vi "401_Add_Inspection_Audit_Data.vi"(0 "Current":variant, 1 "Previous":variant, 3 "Tolerance":u16(ring) items=["Area", "Width", "Height", "Spot", "Color", "Crack", "Foreign Particle", "Foreign outside Pocket"], 4 "Filter":u16(ring) items=["Area", "Width", "Height", "Smooth", "Solid"], 5 "Count":u16(ring) items=["Blister", "Blister 2", "OCV", "Splice 1", "Splice 2", "Pinhole 1", "Pinhole 2", "Spare Sensor 1", "Sealing", "OverPrinting", "Perforation", "Forming"], 7 "Error":errorcluster, 8 "Count/#Rej":string, 9 "Min/Max":string, 10 "Action":T1(ring), 11 "FilterMax/Min":string, 12 "Color":u16(ring) items=["Color 1", "Color 2"]) -> (27 "error out":errorcluster)   [LabVIEW 2015]
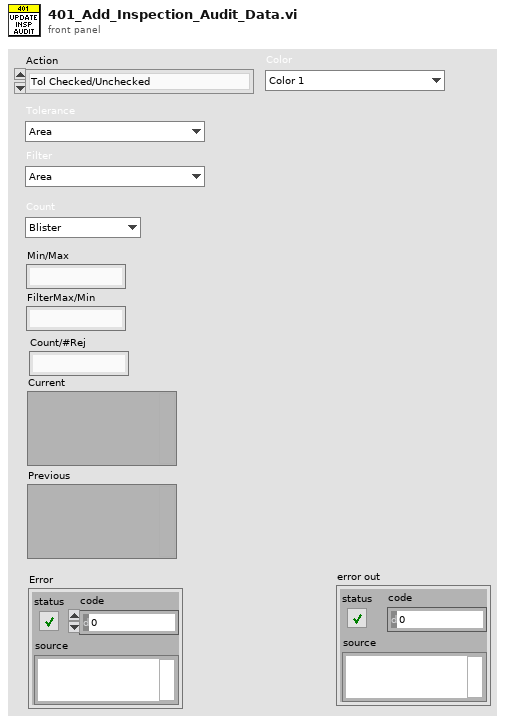
[diagram p1: front panel]
types:
  T1 = enum16{"Tol Checked/Unchecked", "Filter Checked/Unchecked", "Count Value updated", "Tol Updated", "Filter Updated"}
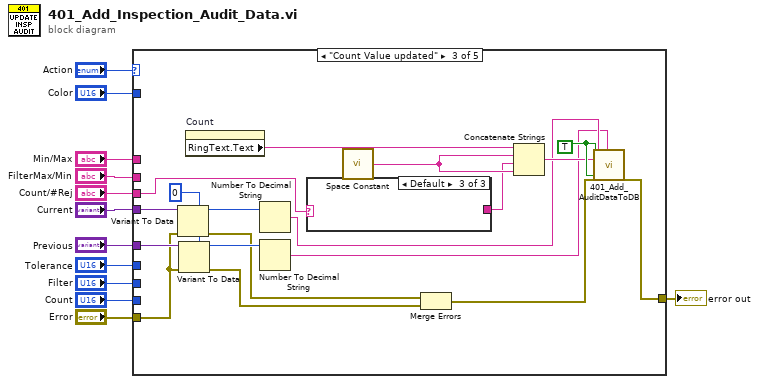
[diagram p0: block diagram]
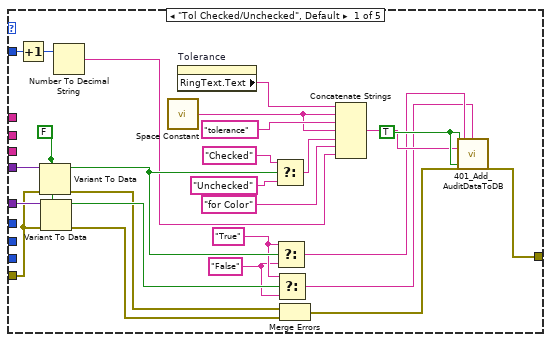
[diagram p2: hidden frame]
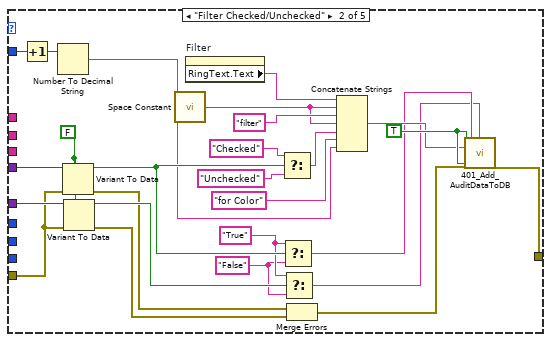
[diagram p3: hidden frame]
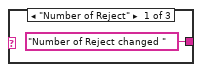
[diagram p4: hidden frame]
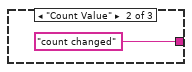
[diagram p5: hidden frame]
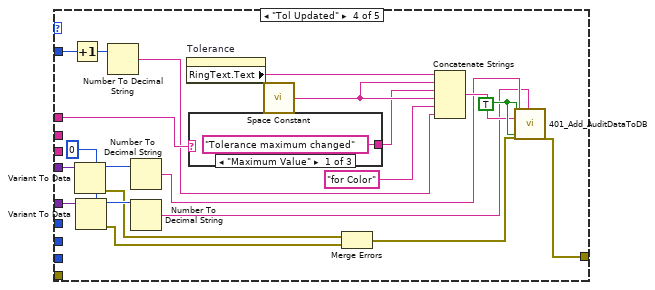
[diagram p6: hidden frame]
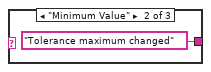
[diagram p7: hidden frame]
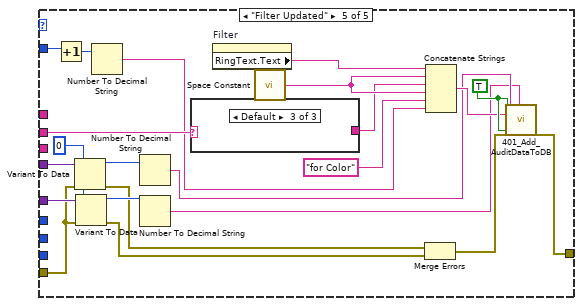
[diagram p9: hidden frame]
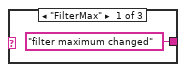
[diagram p10: hidden frame]
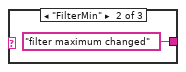
[diagram p11: hidden frame]
diagram:
  n1 = case shown="\"Count Value updated\"" "Action" {
    tunnel: "Current" -> [w38 w49 w78 w94 w118]
    tunnel: "Previous" -> [w37 w48 w77 w95 w119]
    tunnel: "Tolerance" -> [_ _ _ _ _]
    tunnel: "Filter" -> [_ _ _ _ _]
    tunnel: "Count" -> [_ _ _ _ _]
    tunnel: "FilterMax/Min" -> [_ _ _ _ w117]
    tunnel: "Min/Max" -> [_ _ _ w93 _]
    tunnel: "Error" -> [w21 w45 w70 _ w116]
    tunnel: [w17 w47 w66 w89 w112] -> w3
    tunnel: "Count/#Rej" -> [_ _ w65 _ _]
    tunnel: "Color" -> [w16 w41 _ w87 w109]
    frame "Tol Checked/Unchecked", Default {
      w24 = "False" ("string")
      w25 = "True" ("string")
      w29 = TRUE ("str(T)/num")
      w36 = FALSE
      n2 = Increment(x=w16) -> (x+1=w15:u16)
      n3 = Variant To Data(error in=w21, type=w36, Variant=w38) -> (data=w27:bool, error out=w19:errorcluster)
      n4 = Variant To Data(error in=w21, type=w36, Variant=w37) -> (data=w26:bool, error out=w18:errorcluster)
      n5 = Number To Decimal String(number=w15) -> (decimal integer string=w14:string)  [unwired: 1 in]
      n6 = call <vilib>:"Space Constant.vi"() -> ("String"=w33:string)
      n7 = property on="Tolerance" class="Ring (strict)"() -> ("RingText.Text"=w35:string)  [unwired: 2 in, 2 out]
      n8 = Select(t="Checked" ("string"), s=w27, f="Unchecked" ("string")) -> (s? t:f=w30:string)
      n9 = Select(t=w25, s=w27, f=w24) -> (s? t:f=w23:string)
      n10 = Select(t=w25, s=w26, f=w24) -> (s? t:f=w22:string)
      n11 = Merge Errors(w19, w18) -> (w20:errorcluster)
      n12 = Concatenate Strings(w35, w33, "tolerance" ("string"), w33, w30, "for Color" ("string"), w14) -> (w28:string)
      n13 = call "401_Add_AuditDataToDB.vi"("Str(T)/Num"=w29, "Activity"=w28, "Enum(F)/Str"=w29, "error in (no error)"=w20, "Current Value"=w23, "Previous Value"=w22) -> ("error out"=w17:errorcluster)  [unwired: 21 in]
    }
    frame "Filter Checked/Unchecked" {
      w52 = "False" ("string")
      w53 = "True" ("string")
      w57 = TRUE ("str(T)/num")
      w64 = FALSE
      n14 = Increment(x=w41) -> (x+1=w42:u16)
      n15 = Number To Decimal String(number=w42) -> (decimal integer string=w39:string)  [unwired: 1 in]
      n16 = Variant To Data(error in=w45, type=w64, Variant=w49) -> (data=w55:bool, error out=w44:errorcluster)
      n17 = Variant To Data(error in=w45, type=w64, Variant=w48) -> (data=w54:bool, error out=w43:errorcluster)
      n18 = call <vilib>:"Space Constant.vi"() -> ("String"=w61:string)
      n19 = property on="Filter" class="Ring (strict)"() -> ("RingText.Text"=w63:string)  [unwired: 2 in, 2 out]
      n20 = Select(t="Checked" ("string"), s=w55, f="Unchecked" ("string")) -> (s? t:f=w58:string)
      n21 = Select(t=w53, s=w55, f=w52) -> (s? t:f=w51:string)
      n22 = Select(t=w53, s=w54, f=w52) -> (s? t:f=w50:string)
      n23 = Merge Errors(w44, w43) -> (w46:errorcluster)
      n24 = Concatenate Strings(w63, w61, "filter" ("string"), w61, w58, "for Color" ("string"), w39) -> (w56:string)
      n25 = call "401_Add_AuditDataToDB.vi"("Str(T)/Num"=w57, "Activity"=w56, "Enum(F)/Str"=w57, "error in (no error)"=w46, "Current Value"=w51, "Previous Value"=w50) -> ("error out"=w47:errorcluster)  [unwired: 21 in]
    }
    frame "Count Value updated" {
      w76 = 0 ("Previous Value")
      w80 = TRUE ("str(T)/num")
      n26 = Variant To Data(error in=w70, type=w76, Variant=w78) -> (data=w75:i32, error out=w69:errorcluster)
      n27 = Variant To Data(error in=w70, type=w76, Variant=w77) -> (data=w73:i32, error out=w68:errorcluster)
      n28 = property on="Count" class="Ring (strict)"() -> ("RingText.Text"=w82:string)  [unwired: 2 in, 2 out]
      n29 = Number To Decimal String(number=w75) -> (decimal integer string=w72:string)  [unwired: 1 in]
      n30 = Number To Decimal String(number=w73) -> (decimal integer string=w71:string)  [unwired: 1 in]
      n31 = case shown="Default" w65 {
        tunnel: ["Number of Reject changed " ("string") "count changed" ("string") _] -> w74
        frame "Number of Reject" {
        }
        frame "Count Value" {
        }
        frame Default {
        }
      }
      n32 = call <vilib>:"Space Constant.vi"() -> ("String"=w81:string)
      n33 = Merge Errors(w69, w68) -> (w67:errorcluster)
      n34 = Concatenate Strings(w82, w81, w74, w81) -> (w79:string)
      n35 = call "401_Add_AuditDataToDB.vi"("Str(T)/Num"=w80, "Activity"=w79, "Enum(F)/Str"=w80, "error in (no error)"=w67, "Current Value"=w72, "Previous Value"=w71) -> ("error out"=w66:errorcluster)  [unwired: 21 in]
    }
    frame "Tol Updated" {
      w101 = 0 ("Previous Value")
      w103 = TRUE ("str(T)/num")
      n36 = Increment(x=w87) -> (x+1=w88:u16)
      n37 = Variant To Data(type=w101, Variant=w94) -> (data=w100:i32, error out=w92:errorcluster)  [unwired: 1 in]
      n38 = Variant To Data(type=w101, Variant=w95) -> (data=w98:i32, error out=w91:errorcluster)  [unwired: 1 in]
      n39 = Number To Decimal String(number=w88) -> (decimal integer string=w86:string)  [unwired: 1 in]
      n40 = Number To Decimal String(number=w100) -> (decimal integer string=w97:string)  [unwired: 1 in]
      n41 = Number To Decimal String(number=w98) -> (decimal integer string=w96:string)  [unwired: 1 in]
      n42 = property on="Tolerance" class="Ring (strict)"() -> ("RingText.Text"=w105:string)  [unwired: 2 in, 2 out]
      n43 = case shown="\"Maximum Value\"" w93 {
        tunnel: ["Tolerance maximum changed" ("string") "Tolerance maximum changed" ("string") _] -> w99
        frame "Maximum Value" {
        }
        frame "Minimum Value" {
        }
        frame Default {
        }
      }
      n44 = call <vilib>:"Space Constant.vi"() -> ("String"=w104:string)
      n45 = Merge Errors(w92, w91) -> (w90:errorcluster)
      n46 = Concatenate Strings(w105, w104, w99, w104, "for Color" ("string"), w86) -> (w102:string)
      n47 = call "401_Add_AuditDataToDB.vi"("Str(T)/Num"=w103, "Activity"=w102, "Enum(F)/Str"=w103, "error in (no error)"=w90, "Current Value"=w97, "Previous Value"=w96) -> ("error out"=w89:errorcluster)  [unwired: 21 in]
    }
    frame "Filter Updated" {
      w125 = 0 ("Previous Value")
      w127 = TRUE ("str(T)/num")
      n48 = Increment(x=w109) -> (x+1=w110:u16)
      n49 = Variant To Data(error in=w116, type=w125, Variant=w118) -> (data=w124:i32, error out=w114:errorcluster)
      n50 = Variant To Data(error in=w116, type=w125, Variant=w119) -> (data=w122:i32, error out=w113:errorcluster)
      n51 = Number To Decimal String(number=w110) -> (decimal integer string=w108:string)  [unwired: 1 in]
      n52 = Number To Decimal String(number=w124) -> (decimal integer string=w121:string)  [unwired: 1 in]
      n53 = Number To Decimal String(number=w122) -> (decimal integer string=w120:string)  [unwired: 1 in]
      n54 = case shown="Default" w117 {
        tunnel: ["filter maximum changed" ("string") "filter maximum changed" ("string") _] -> w123
        frame "FilterMax" {
        }
        frame "FilterMin" {
        }
        frame Default {
        }
      }
      n55 = property on="Filter" class="Ring (strict)"() -> ("RingText.Text"=w129:string)  [unwired: 2 in, 2 out]
      n56 = call <vilib>:"Space Constant.vi"() -> ("String"=w128:string)
      n57 = Merge Errors(w114, w113) -> (w115:errorcluster)
      n58 = Concatenate Strings(w129, w128, w123, w128, "for Color" ("string"), w108) -> (w126:string)
      n59 = call "401_Add_AuditDataToDB.vi"("Str(T)/Num"=w127, "Activity"=w126, "Enum(F)/Str"=w127, "error in (no error)"=w115, "Current Value"=w121, "Previous Value"=w120) -> ("error out"=w112:errorcluster)  [unwired: 21 in]
    }
  }
  "error out" <- w3
